vi "被反馈处理.vi"(0 "识别名称":string, 2 "校验信息":cluster{"可用？":bool, "功能码":u8, "无crc报文":u8[]}, 10 "等待时间（毫秒）":u32) -> (14 "识别名称输出":string, 15 "反馈":string)   [LabVIEW 2019]
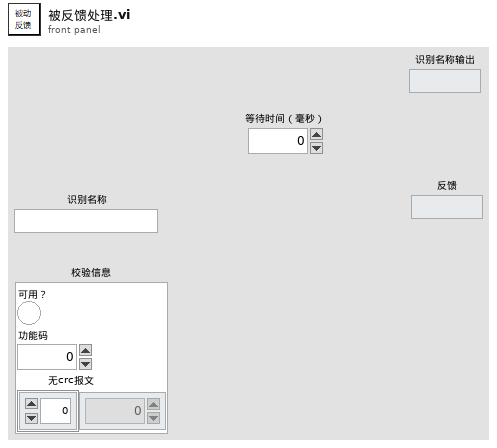
[diagram p1: front panel]
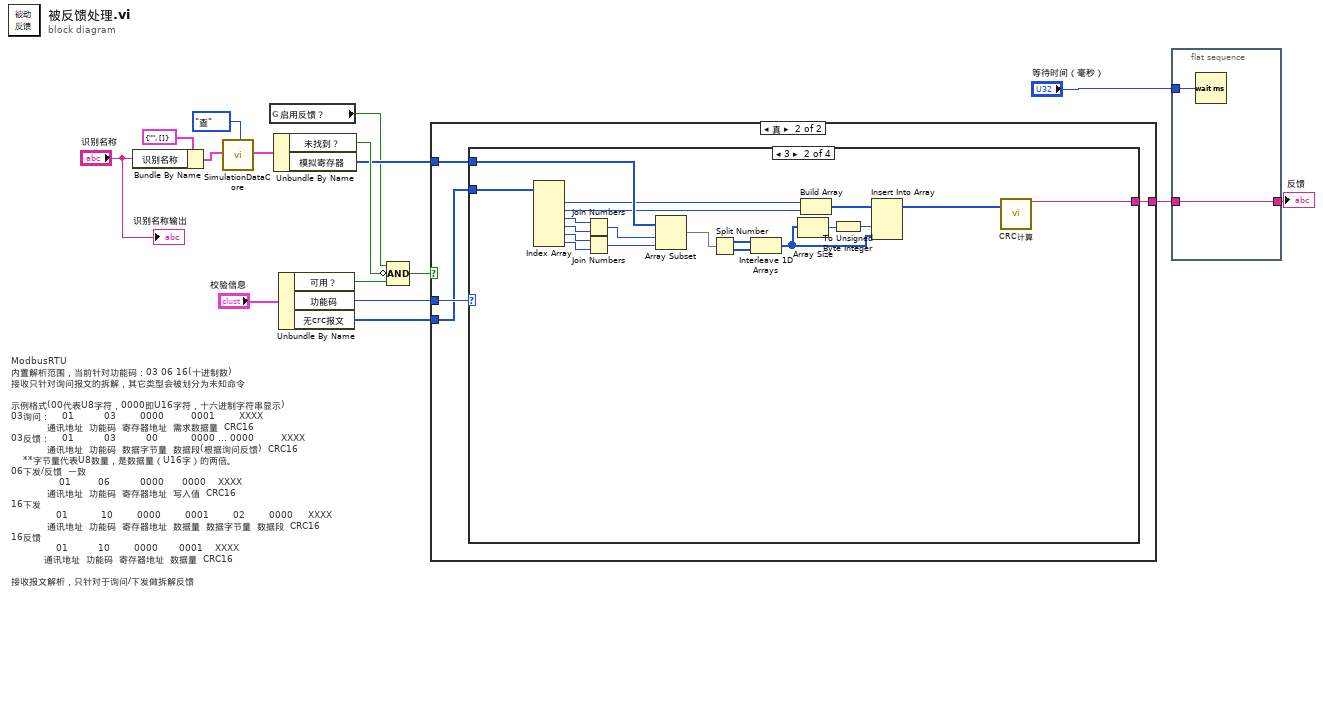
[diagram p0: block diagram]
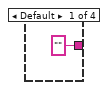
[diagram p3: hidden frame]
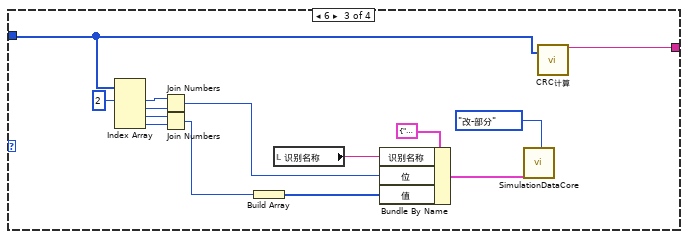
[diagram p4: hidden frame]
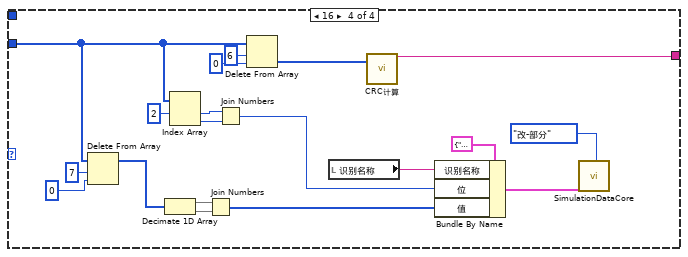
[diagram p5: hidden frame]
diagram:
  # "ModbusRTU\n内置解析范围，当前针对功能码：03 06 16(十进制数)\n接收只针对询问报文的拆解，其它类型会被划分为未知命令\n\n示例格式(00代表U8字符，0000即U16字符，十六进制字符串显示)\n03询问：    01          03        0000         0001        XXXX \n            通讯地址  功能码  寄存器地址  需求数据量  CRC16\n03反馈：    01          03          00           0000 ... 0000         XXXX \n            通讯地址  功能码  数据字节量  数据段(根据询问反馈)  CRC16\n    **字节量代表U8数量，是数据量（U16字）的两倍。\n06下发/反馈  一致\n                01         06          0000      0000    XXXX\n            通讯地址  功能码  寄存器地址  写入值  CRC16\n16下发\n               01           10        0000        0001        02        0000     XXXX\n            通讯地址  功能码  寄存器地址  数据量  数据字节量  数据段  CRC16 \n16反馈\n               01          10        0000       0001    XXXX\n           通讯地址  功能码  寄存器地址  数据量  CRC16\n\n接收报文解析，只针对于询问/下发做拆解反馈"
  n1 = Bundle By Name(cluster=cluster{"识别名称":string, "模拟寄存器":u16[]} {"识别名称"="", "模拟寄存器"=[]} ("配置信息"), "识别名称"="识别名称") -> (w14:cluster{"识别名称":string, "模拟寄存器":u16[]})
  n2 = call "SimulationDataCore.vi"("配置信息"=w14, "模拟数据枚举"=enum16{"ini", "增", "删", "查", "改-全", "改-部分"}."查") -> ("结果"=w13:cluster{"未找到？":bool, "模拟寄存器":u16[]})  [unwired: 16 in, 1 out]
  n3 = global read "全局-被反馈配置.vi" "启用反馈？"() -> (w4:bool)
  n4 = Unbundle By Name(w13) -> ("未找到？"=w8:bool, "模拟寄存器"=w6:u16[])
  n5 = Unbundle By Name("校验信息") -> ("可用？"=w9:bool, "功能码"=w11:u8, "无crc报文"=w10:u8[])
  n6 = Compound Arithmetic op=AND ("复合运算")(w4, invert w8, w9) -> (w7:bool)
  n7 = case shown="真" w7 {
    tunnel: w11 -> [_ w20]
    tunnel: w10 -> [_ w19]
    tunnel: w6 -> [_ w18]
    tunnel: [_ w17] -> w3
    frame False {
    }
    frame True {
      n8 = case shown="3" w20 {
        tunnel: w19 -> [_ w40 w53 w60]
        tunnel: w18 -> [_ w35 _ _]
        tunnel: ["" ("计算后字符串") w22 w52 w56] -> w17
        frame Default {
        }
        frame 3 {
          n9 = Index Array(array=w40) -> (element #1=w32:u8, element #2=w31:u8, element #3=w39:u8, element #4=w38:u8, element #5=w37:u8, element #6=w36:u8)  [unwired: 6 in]
          n10 = Join Numbers(hi=w39, lo=w38) -> ((hi.lo)=w34:u16)
          n11 = Join Numbers(hi=w37, lo=w36) -> ((hi.lo)=w33:u16)
          n12 = Array Subset(array=w35, index=w34, length=w33) -> (w25:u16[])
          n13 = Split Number(x=w25) -> (hi(x)=w27:u8[], lo(x)=w26:u8[])
          n14 = Interleave 1D Arrays(w27, w26) -> (w24:u8[])
          n15 = Array Size(array=w24) -> (size(s)=w29:i32)
          n16 = Build Array(w32, w31) -> (w30:u8[])
          n17 = To Unsigned Byte Integer(number=w29) -> (unsigned 8bit integer=w28:u8)
          n18 = Insert Into Array(array=w30, new element #1=w28, new element #2=w24) -> (w23:u8[])  [unwired: 1 in]
          n19 = call "CRC计算.vi"("无校验U8数组"=w23) -> ("计算后字符串"=w22:string)  [unwired: 17 in, 1 out]
        }
        frame 6 {
          n20 = Index Array(array=w53, index #1=2 ("索引")) -> (element #1=w51:u8, element #2=w50:u8, element #3=w49:u8, element #4=w48:u8)  [unwired: 3 in]
          n21 = Join Numbers(hi=w51, lo=w50) -> ((hi.lo)=w43:u16)
          n22 = Join Numbers(hi=w49, lo=w48) -> ((hi.lo)=w42:u16)
          n23 = Build Array(w42) -> (w41:u16[])
          n24 = local read "识别名称"() -> (w44:string)
          n25 = Bundle By Name(cluster=cluster{"识别名称":string, "位":u16, "值":u16[]} {"识别名称"="", "位"=0, "值"=[]} ("改部分配置"), "识别名称"=w44, "位"=w43, "值"=w41) -> (w45:cluster{"识别名称":string, "位":u16, "值":u16[]})
          n26 = call "SimulationDataCore.vi"("改部分配置"=w45, "模拟数据枚举"=enum16{"ini", "增", "删", "查", "改-全", "改-部分"}."改-部分") -> ()  [unwired: 16 in, 2 out]
          n27 = call "CRC计算.vi"("无校验U8数组"=w53) -> ("计算后字符串"=w52:string)  [unwired: 17 in, 1 out]
        }
        frame 16 {
          n28 = Delete From Array(array=w60, length=7 ("长度"), index=0 ("索引")) -> (array with subset deleted=w63:u8[])  [unwired: 1 out]
          n29 = Decimate 1D Array(w63) -> (w62:u8[], w61:u8[])
          n30 = Index Array(array=w60, index #1=2 ("索引")) -> (element #1=w73:u8, element #2=w72:u8)  [unwired: 1 in]
          n31 = Join Numbers(hi=w62, lo=w61) -> ((hi.lo)=w55:u16[])
          n32 = Join Numbers(hi=w73, lo=w72) -> ((hi.lo)=w69:u16)
          n33 = Delete From Array(array=w60, length=6 ("长度"), index=0 ("索引")) -> (deleted portion=w57:u8[])  [unwired: 1 out]
          n34 = local read "识别名称"() -> (w70:string)
          n35 = call "CRC计算.vi"("无校验U8数组"=w57) -> ("计算后字符串"=w56:string)  [unwired: 17 in, 1 out]
          n36 = Bundle By Name(cluster=cluster{"识别名称":string, "位":u16, "值":u16[]} {"识别名称"="", "位"=0, "值"=[]} ("改部分配置"), "识别名称"=w70, "位"=w69, "值"=w55) -> (w71:cluster{"识别名称":string, "位":u16, "值":u16[]})
          n37 = call "SimulationDataCore.vi"("改部分配置"=w71, "模拟数据枚举"=enum16{"ini", "增", "删", "查", "改-全", "改-部分"}."改-部分") -> ()  [unwired: 16 in, 2 out]
        }
      }
    }
  }
  n38 = flat-sequence {
    tunnel: w3 -> [w75]
    tunnel: [w75] -> w2
    tunnel: "等待时间（毫秒）" -> [w74]
    frame #0 {
      n39 = Wait (ms)(milliseconds to wait=w74) -> ()  [unwired: 1 out]
    }
  }
  "反馈" <- w2
  "识别名称输出" <- "识别名称"
